vi "UI_Frequency_Settings.vi"() -> ()   [LabVIEW 2014]
panel:
  in  "退出":bool
  in  "保存":bool
  in  "表格控件":string[][](table)
  # "采样频率设置"
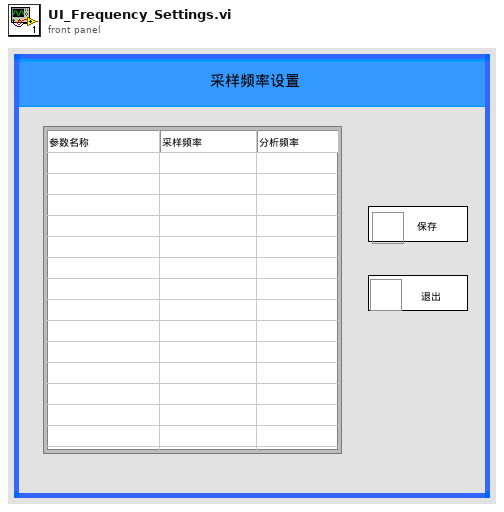
[diagram p1: front panel]
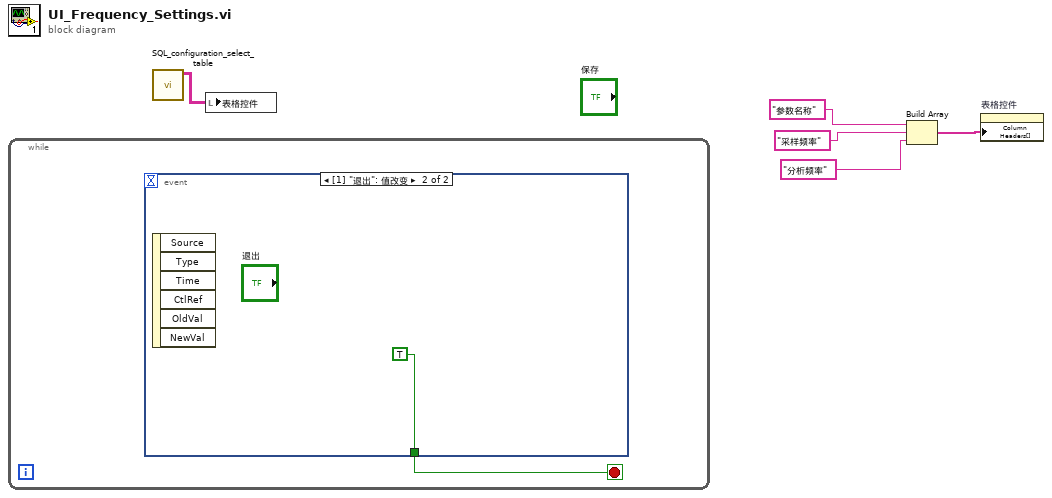
[diagram p0: block diagram]
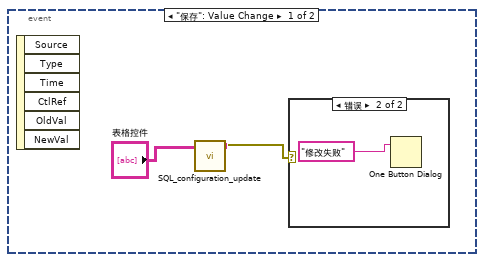
[diagram p2: hidden frame]
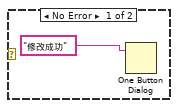
[diagram p3: hidden frame]
diagram:
  n1 = while {
    stop <- w6 stop-if-true
    n2 = event shown="[1] \"退出\": 值改变" {
      selector: _ -> [_ _]
      dyn-events: _ -> [_ _]
      timeout: _ -> [_ _]
      tunnel: [_ TRUE] -> w6
      event "保存": Value Change {
        n3 = event-data() -> ()  [unwired: 1 in, 6 out]
        n4 = call "SQL_configuration_update.vi"("表格控件"="表格控件") -> ("error out"=w7:errorcluster)  [unwired: 10 in]
        n5 = case shown="错误" w7 {
          frame No Error {
            n6 = One Button Dialog(message="修改成功") -> ()  [unwired: 1 in, 1 out]
          }
          frame Error {
            n7 = One Button Dialog(message="修改失败") -> ()  [unwired: 1 in, 1 out]
          }
        }
      }
      event "退出": Value Change {
        n8 = event-data() -> ()  [unwired: 1 in, 6 out]
      }
    }
  }
  n9 = call "SQL_configuration_select_table.vi"() -> ("表格控件"=w1:string[][])  [unwired: 10 in, 1 out]
  n10 = local write "表格控件"(w1) -> ()
  n11 = Build Array("参数名称", "采样频率", "分析频率") -> (w2:string[])
  n12 = property on="表格控件" class="Tbl (严格)"("Column Headers[]"=w2) -> ()  [unwired: 2 in, 2 out]
